vi "Temperature Monitor (Demo).vi3-4.vi"() -> ()   [LabVIEW 2014]
doc: "This VI is the solution to an exercise in the LabVIEW Core I course.\n\nIt is used to demonstrate While loops and waveform charts. This VI simulates a temperature reading once every 500 ms and plots the data in a strip chart."
panel:
  out "Temperature History":dbl(graph)
  in  "Power":bool=TRUE
  # "ON\n\nOFF"
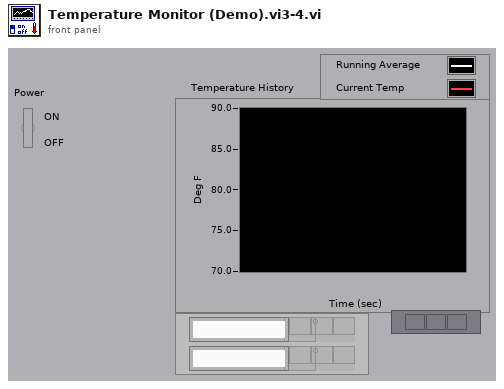
[diagram p1: front panel]
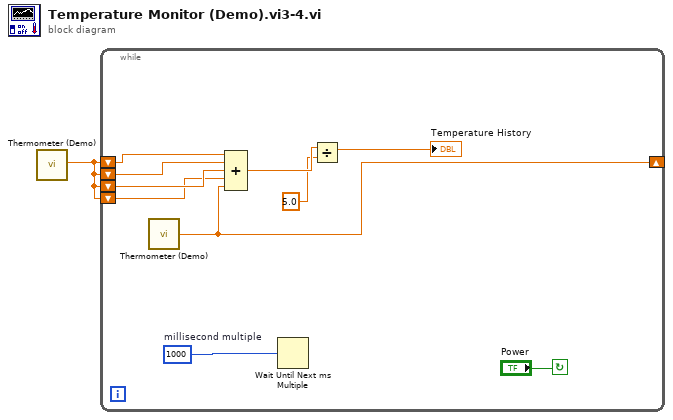
[diagram p0: block diagram]
diagram:
  n1 = call "Thermometer (Demo).vi"() -> ("Temperature"=w1:dbl)  [unwired: 1 in]
  n2 = while {
    shift-right: [w2] -> _
    shift-left: w1 -> [w9]
    shift-left: w1 -> [w7]
    shift-left: w1 -> [w8]
    shift-left: w1 -> [w6]
    stop <- "Power" continue-if-true
    w10 = u32 1000  # millisecond multiple
    n3 = call "Thermometer (Demo).vi"() -> ("Temperature"=w2:dbl)  [unwired: 1 in]
    n4 = Compound Arithmetic op=ADD(w9, w8, w7, w6, w2) -> (w5:dbl)
    n5 = Wait Until Next ms Multiple(millisecond multiple=w10) -> ()  [unwired: 1 out]
    n6 = Divide(x=w5, y=5.0) -> (x/y=→"Temperature History":dbl)
  }
